vi "5.3 Cluster 2D Array to CSM API String.vi"() -> ()   [LabVIEW 2017]
doc: "#### Overview\n\nDemonstrates API String expression for 2-D array of clusters.\n\n#### Introduction\n\nAn array is a composite data type that may contain different data types, with cluster being the most complex. This example shows the API String expression for 2-D array of clusters."
uses:
  9f1c8977-aa41-4596-a18a-6dba2ebc59d2.vi
  0333efe5-f0fb-4901-b6dd-db031cec30c6.vi
  addons/API-String-Arugments-Support/_Support/Data To API String Arguments.vi
  addons/API-String-Arugments-Support/_Support/Convert API String Arguments to Data(variant).vi
panel:
  out "String":string
  in  "Array":T1(array[cluster])=[[{"String"="abc", "BoolArray"=[[TRUE, FALSE, TRUE, FALSE], [FALSE, TRUE, FALSE, TRUE], [TRUE, FALSE, TRUE, FALSE]], "Boolean"=FALSE}, {"String"="def", "BoolArray"=[[TRUE, FALSE, TRUE, FALSE], [FALSE, TRUE, FALSE, TRUE], [TRUE, FALSE, TRUE, FALSE]], "Boolean"=TRUE}], [{"String"="123", "BoolArray"=[[FALSE, FALSE, TRUE, FALSE], [FALSE, TRUE, FALSE, TRUE], [TRUE, TRUE, TRUE, FALSE]], "Boolean"=TRUE}, {"String"="456", "BoolArray"=[[TRUE, TRUE, TRUE, FALSE], [TRUE, FALSE, FALSE, TRUE], [FALSE, FALSE, TRUE, FALSE]], "Boolean"=FALSE}]]
  out "Array":T1(array[cluster])=[[{"String"="abc", "BoolArray"=[[TRUE, FALSE, TRUE, FALSE], [FALSE, TRUE, FALSE, TRUE], [TRUE, FALSE, TRUE, FALSE]], "Boolean"=FALSE}, {"String"="def", "BoolArray"=[[TRUE, FALSE, TRUE, FALSE], [FALSE, TRUE, FALSE, TRUE], [TRUE, FALSE, TRUE, FALSE]], "Boolean"=TRUE}]]
  # "#CSM-Example Overview\n\nDemonstrates API String expression for 2-D array of clusters."
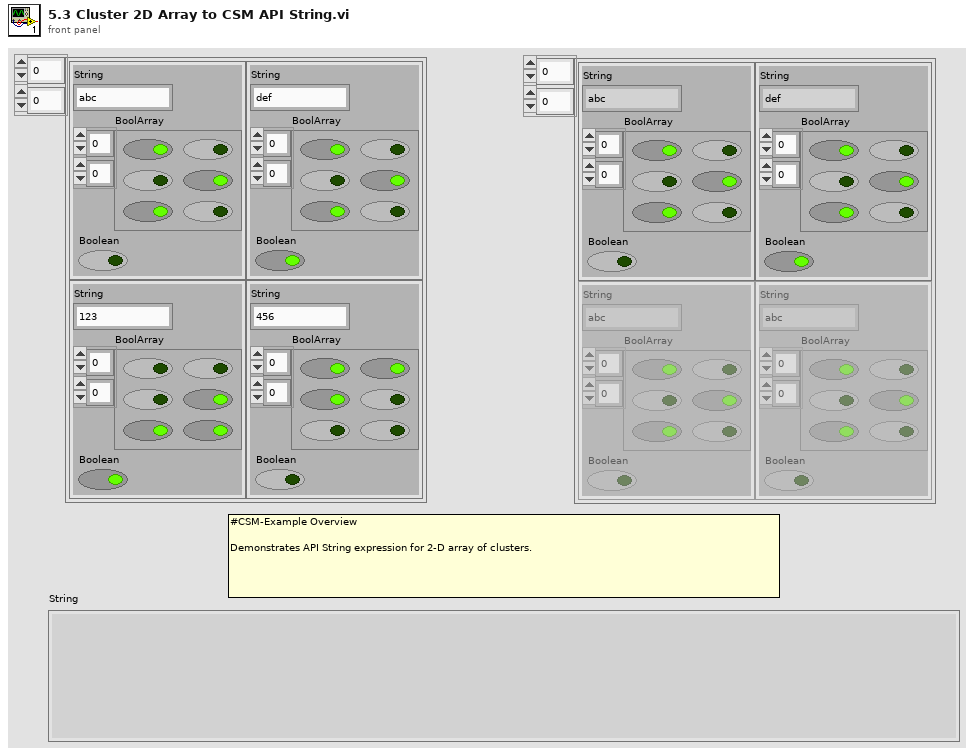
[diagram p1: front panel]
types:
  T1 = cluster{"String":string, "BoolArray":bool[][], "Boolean":bool}[][]
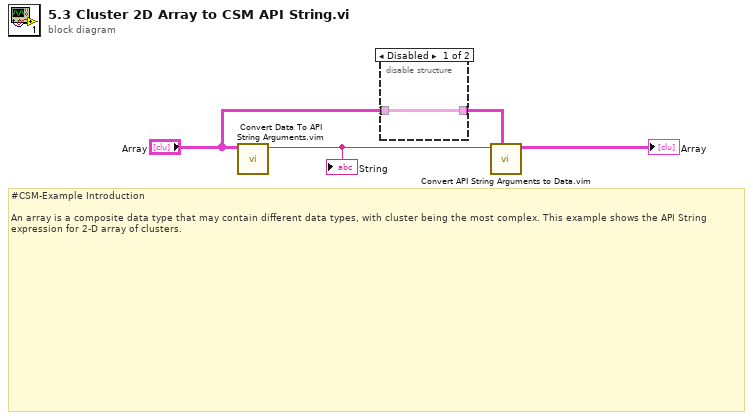
[diagram p0: block diagram]
diagram:
  # "#CSM-Example Introduction\n\nAn array is a composite data type that may contain different data types, with cluster being the most complex. This example shows the API String expression for 2-D array of clusters."
  n1 = call "Convert Data To API String Arguments.vim"("Data"="Array") -> ("API String"=w1:string)  [unwired: 7 in, 1 out]
  "String" <- w1
  n2 = disable-structure "Diagram Disable Structure" shown="Disabled" {
    disable-tunnel: "Array" -> [w5 _]
    disable-tunnel: [w5 _] -> w3
    frame Disabled {
    }
    frame Enabled {
    }
  }
  n3 = call "Convert API String Arguments to Data.vim"("Reference Type"=w3, "API String"=w1) -> ("Data"=→"Array":T1)  [unwired: 6 in, 1 out]
